vi "New.vi"(6 "Configuration":string, 7 "Class Manager Reference":refnum<data-value>, 8 "error in (no error)":errorcluster, 10 "Name":string, 11 "Child Class in":refnum<class "Instrument.lvclass">) -> (0 "error out":errorcluster, 3 "Child Class out":refnum<class "Instrument.lvclass">)   [LabVIEW 2017, in "Instrument.lvlib" / "Instrument.lvclass"]
uses:
  Instrument.lvclass
  <vilib>/TSS/ACRObat Test Framework/Classes/Class Register/Class Register.lvclass
  Properties/Instrument Properties.lvclass
  Instrument.lvclass/Instrument.ctl
  <vilib>/TSS/ACRObat Test Framework/Classes/Base Objects/Acrobat Base Object/Acrobat Base Object/Acrobat Base Object.lvclass
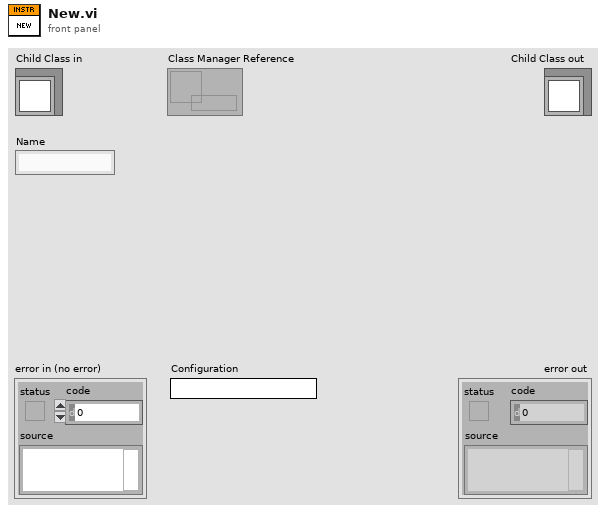
[diagram p1: front panel]
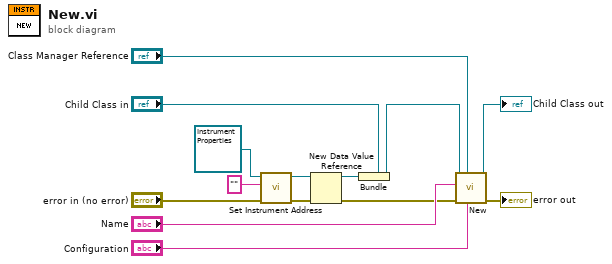
[diagram p0: block diagram]
diagram:
  n1 = call-dynamic "Set Instrument Address.vi"("error in (no error)"="error in (no error)", "Instrument Address"="", "Instrument Properties in"=refnum<class "Instrument Properties.lvclass"> refnum) -> ("error out"=w5:errorcluster, "Instrument Properties out"=w3:refnum<class "Instrument Properties.lvclass">)  [unwired: 7 in]
  n2 = New Data Value Reference(data value=w3, error in=w5) -> (data value reference=w1:refnum<data-value>, error out=w4:errorcluster)
  n3 = Bundle(cluster="Child Class in", w1) -> (w6:refnum<class "Instrument.lvclass">)
  n4 = call-parent "New.vi"("Configuration"="Configuration", "Class Manager Reference"="Class Manager Reference", "error in (no error)"=w4, "Name"="Name", "Child Class in"=w6) -> ("error out"=→"error out":errorcluster, "Child Class out"=→"Child Class out":refnum<class "Instrument.lvclass">)  [unwired: 5 in]
